vi "Untitled 1.vi"() -> ()   [LabVIEW 2017]
uses:
  Users/huijun.guo/Desktop/Control_TypeReceiveSeqData.ctl
  <vilib>/gpm_packages/@cs/persistence/source/XML/XML.lvclass
  <vilib>/gpm_packages/@cs/linked-list/Source/String Manipulation/String Manipulation.lvlib
panel:
  out "Array":string[](array[string])
  out "Flattened Test Executive":string[](array[string])
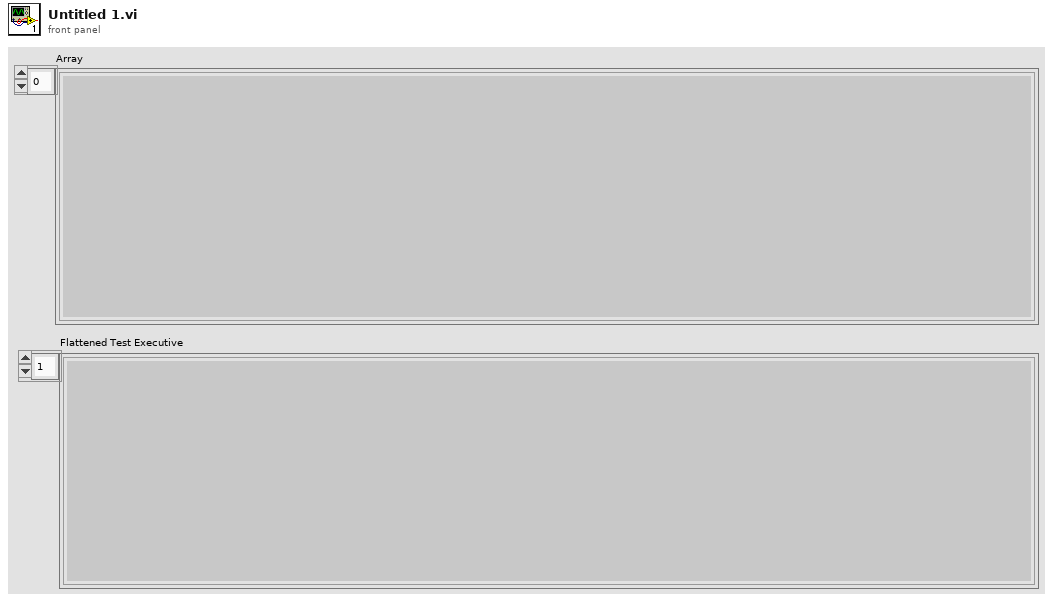
[diagram p1: front panel]
types:
  T1 = typedef "Control_TypeReceiveSeqData.ctl" = cluster{"Slot":enum16{"Slot1", "Slot2", "Slot3", "Slot4", "Slot5", "Slot6", "Slot7", "Slot8", "Slot9", "Slot10", "Slot11", "Slot12", "Slot13", "Slot14", "Slot15", "Slot16", "Slot17", "Slot18", "Slot19", "Slot20", "Slot21", "Slot22", "Slot23", "Slot24", "Slot25", "Slot26", "Slot27", "Slot28", "Slot29", "Slot30", "Slot31", "Slot32"}, "Pass?":bool, "ReturnString":string, "CycleTime":dbl, "StartTimeStamp":timestamp, "EndTimeStamp":timestamp, "RetryCounter":u64, "TestItemIndex":u64, "HighLimit":string, "LowLimit":string, "TestName":string, "Unit":string, "TestEnd?":bool, "AllTestStepPass?":bool, "Action":enum16{"ReturnData", "CMD", "Idle"}, "SaveResult?":bool, "ErrorCode":string, "FlowControl?":enum16{"No", "Yes"}, "SFC":bool, "Serial#":string, "Factory_ID":string, "ProjectName":string, "Build_config":string, "TestDate_Time":string, "Operator":string, "TestStation":string, "Fixture#":string, "Test_Time (sec)":string, "Diag_Ver":string, "ProjectLine":string, "Gui_Ver":string, "Image_Name_Ver":string, "Amazon_HW_Ver":string, "Route_check":string, "More":string}
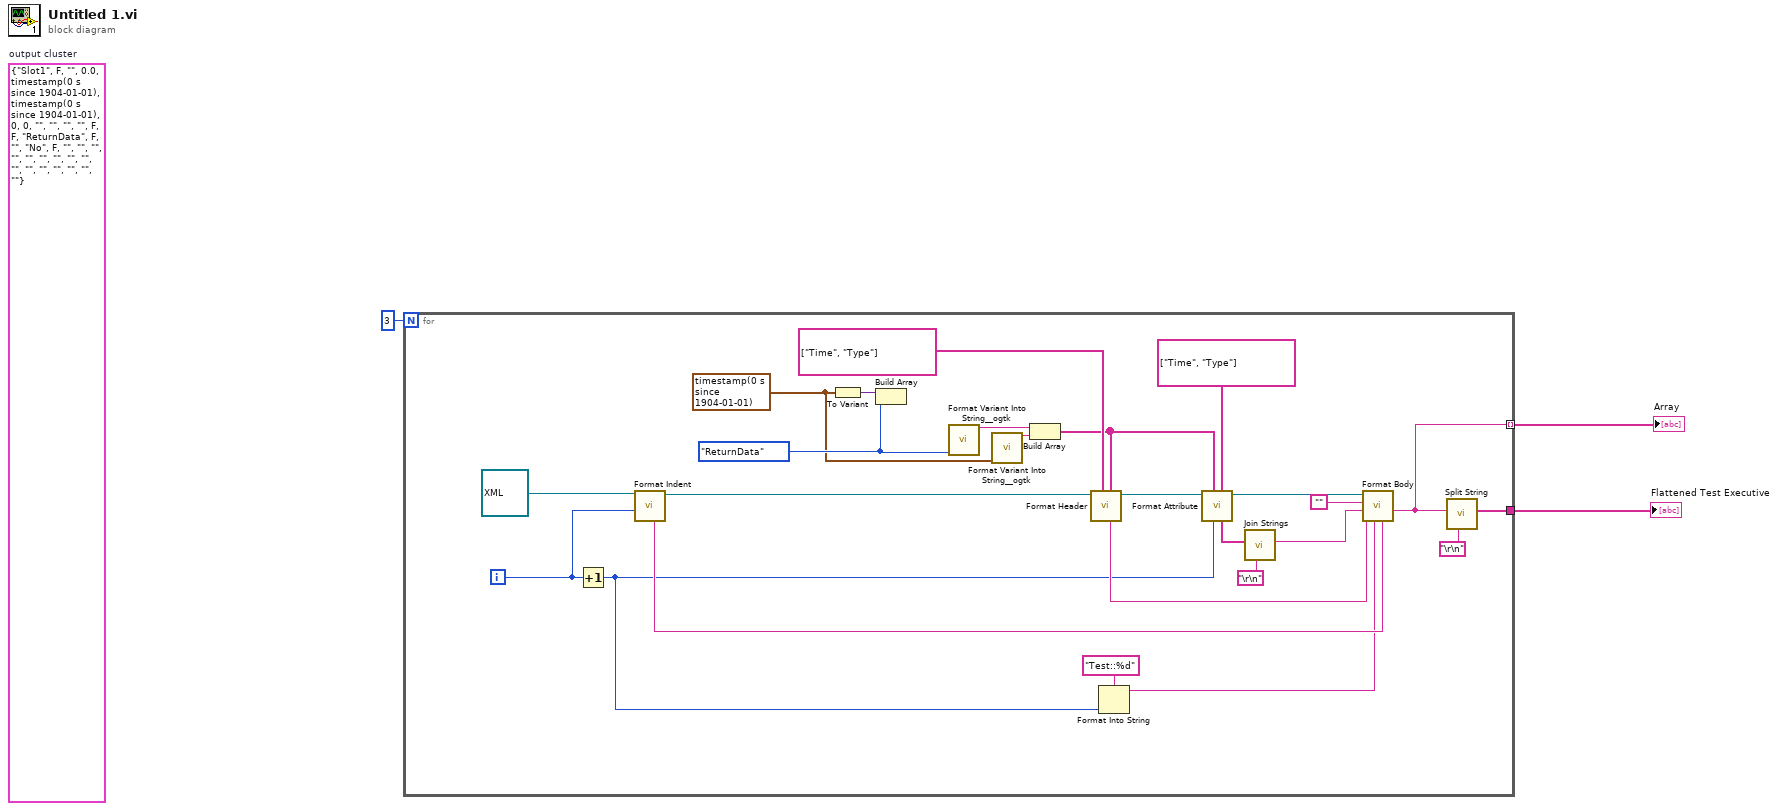
[diagram p0: block diagram]
diagram:
  (unwired) T1 {"Slot"=enum."Slot1", "Pass?"=FALSE, "ReturnString"="", "CycleTime"=0.0, "StartTimeStamp"=timestamp(0 s since 1904-01-01), "EndTimeStamp"=timestamp(0 s since 1904-01-01), "RetryCounter"=0, "TestItemIndex"=0, "HighLimit"="", "LowLimit"="", "TestName"="", "Unit"="", "TestEnd?"=FALSE, "AllTestStepPass?"=FALSE, "Action"=enum."ReturnData", "SaveResult?"=FALSE, "ErrorCode"="", "FlowControl?"=enum."No", "SFC"=FALSE, "Serial#"="", "Factory_ID"="", "ProjectName"="", "Build_config"="", "TestDate_Time"="", "Operator"="", "TestStation"="", "Fixture#"="", "Test_Time (sec)"="", "Diag_Ver"="", "ProjectLine"="", "Gui_Ver"="", "Image_Name_Ver"="", "Amazon_HW_Ver"="", "Route_check"="", "More"=""}  # output cluster
  n1 = for {
    N: 3 -> [_]
    tunnel: [w18] -> w3
    tunnel: [w12] -> w2 mode=indexing
    i -> [w14]
    w7 = timestamp(0 s since 1904-01-01) ("StartTimeStamp")
    w8 = enum16{"ReturnData", "CMD", "Idle"}."ReturnData" ("Action")
    n2 = Increment(x=w14) -> (x+1=w13:i32)
    n3 = call-dynamic "Format Indent.vi"("Indent"=w14, "XML in"=refnum<class "XML.lvclass"> refnum ("XML.lvlib:XML.lvclass")) -> ("XML out"=w28:refnum<class "XML.lvclass">, "Indent XML"=w25:string)  [unwired: 7 in, 1 out]
    n4 = To Variant(anything=w7) -> (Variant=w11:variant)
    n5 = Build Array(w11, w8) -> ()  [unwired: 1 out]
    n6 = call <userlib>:"Format Variant Into String__ogtk.vi"("Variant"=w8) -> ("Output String"=w6:string)  [unwired: 13 in, 1 out]
    n7 = call <userlib>:"Format Variant Into String__ogtk.vi"("Variant"=w7) -> ("Output String"=w5:string)  [unwired: 13 in, 1 out]
    n8 = Build Array(w6, w5) -> (w4:string[])
    n9 = call-dynamic "Format Header.vi"("Name"=w4, "Value"=string[] ["Time", "Type"] ("Attribute Names"), "XML in"=w28) -> ("XML out"=w27:refnum<class "XML.lvclass">, "Header"=w21:string)  [unwired: 7 in]
    n10 = Format Into String(format string="Test::%d", w13) -> (resulting string=w15:string)  [unwired: 2 in, 1 out]
    n11 = call-dynamic "Format Attribute.vi"("Attribute Names"=string[] ["Time", "Type"], "Indent"=w13, "Attribute Values"=w4, "XML in"=w27) -> ("XML out"=w26:refnum<class "XML.lvclass">, "Attr Strings"=w23:string[])  [unwired: 6 in]
    n12 = call <vilib>:"Join Strings.vi"("Separator (,)"="\r\n", "Strings In"=w23) -> ("String"=w22:string)  [unwired: 9 in]
    n13 = call-dynamic "Format Body.vi"("Indent"=w25, "Name"=w15, "Header"=w21, "Attributes"=w22, "Body"="", "XML in"=w26) -> ("String out"=w12:string)  [unwired: 4 in, 1 out]
    n14 = call <vilib>:"Split String.vi"("Split Pattern"="\r\n", "Input String"=w12) -> ("Split String"=w18:string[])  [unwired: 9 in]
  }
  "Flattened Test Executive" <- w3
  "Array" <- w2
